vi "New16bitImage.vi"(8 "error in (no error)":errorcluster, 11 "ImageName":string) -> (0 "error out":errorcluster, 3 "Refnum out":T1)   [LabVIEW 2013, in "GenericCamera.lvclass"]
uses:
  GenericCamera.lvclass
  <vilib>/vision/Image Controls.llb/IMAQ Image.ctl
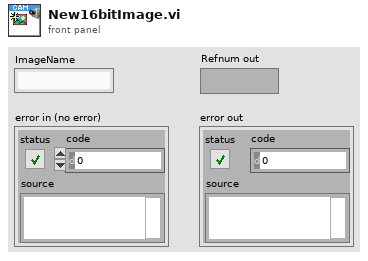
[diagram p1: front panel]
types:
  T1 = typedef "IMAQ Image.ctl" = refnum<image>
  T2 = typedef "Image Type" = u32
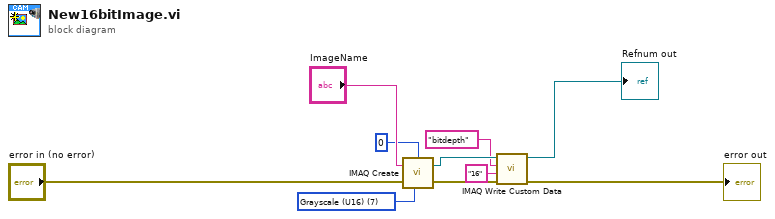
[diagram p0: block diagram]
diagram:
  w3 = T2 7 items=["Grayscale (U8)", "Grayscale (I16)", "Grayscale (SGL)", "Complex (CSG)", "RGB (U32)", "HSL (U32)", "RGB (U64)", "Grayscale (U16)"] ("Image Type")
  n1 = call "IMAQ Create"("Border Size"=0, "Image Name"="ImageName", "Image Type"=w3, "error in (no error)"="error in (no error)") -> ("New Image"=w5:T1, "error out"=w6:errorcluster)  [unwired: 1 in]
  n2 = call "IMAQ Write Custom Data"("error in (no error)"=w6, "Custom Data In"="16", "Key"="bitdepth", "Image"=w5) -> ("error out"=→"error out":errorcluster, "Image Out"=→"Refnum out":T1)  [unwired: 6 in]
